vi "OC2 Read Sensor.vi"(0 "VISA resource name":refnum<visa-resource-name>, 1 "sensor report in":T1 {"Averaging" items=["Off", "On"]; "Unit" items=["deg C", "deg F", "deg K"]; "C coeff." format="%.2f"; "X coeff." format="%.2f"; "X2 coeff." format="%.2f"; "Sensor" items=["None", "PT100", "LM35", "LM50", "LM51", "LM60", "LM61", "Other"]}, 2 "error in (no error)":errorcluster, 5 "Enable":bool) -> (3 "dup VISA resource name":refnum<visa-resource-name>, 4 "sensor report out":T1 {"Averaging" items=["Off", "On"]; "Unit" items=["deg C", "deg F", "deg K"]; "C coeff." format="%.2f"; "X coeff." format="%.2f"; "X2 coeff." format="%.2f"; "Sensor" items=["None", "PT100", "LM35", "LM50", "LM51", "LM60", "LM61", "Other"]}, 6 "error out":errorcluster)   [LabVIEW 2009]
doc: "TCM Read Sensor.vi\n\nVI that reads the sensor information, accepts a cluster that contains the following variables:\nSensor type - PT100, LM35 etc\nx2, x, c coefficients - quadratic equation information\nUnit - unit of measure degrees c, f and kelvin\nAveraging - off no averaging of the signal, on signal is averaged\n\n\nCOPYRIGHT ELECTRON DYNAMICS LTD"
panel:
  in  "Command":string
  out "Rx string":string
  # "Read sensor data"
  # "V1.02"
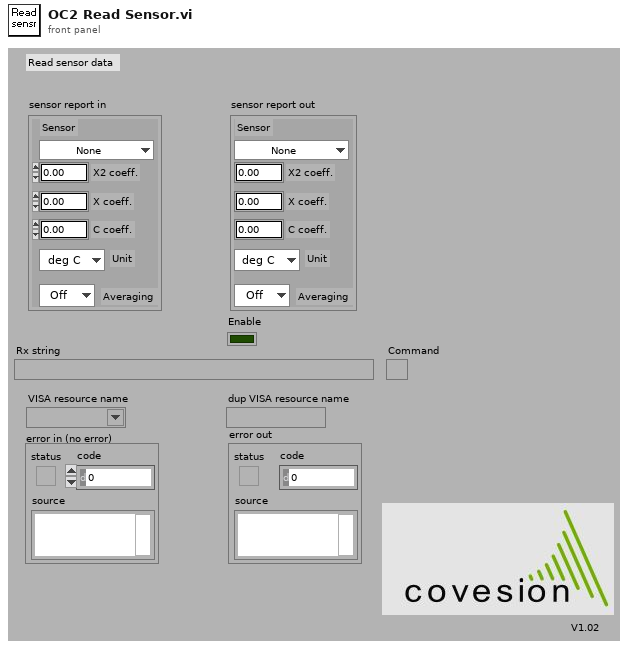
[diagram p1: front panel]
types:
  T1 = cluster{"Sensor":u16, "X2 coeff.":dbl, "X coeff.":dbl, "C coeff.":dbl, "Unit":u16, "Averaging":u16}
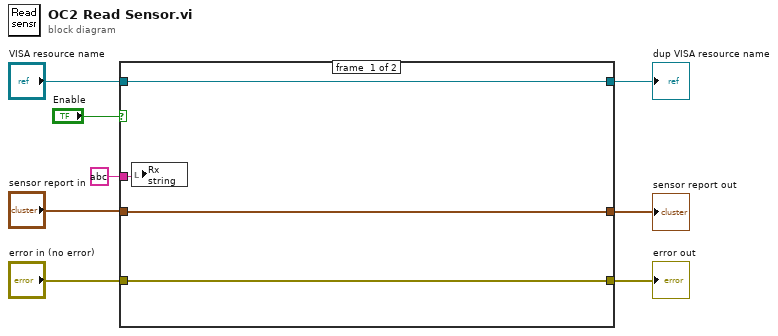
[diagram p0: block diagram]
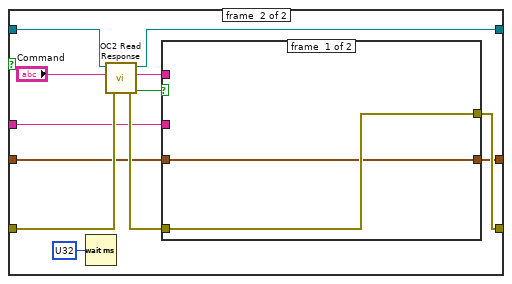
[diagram p2: hidden frame]
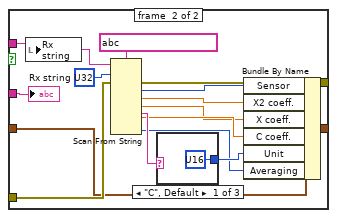
[diagram p3: hidden frame]
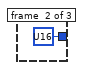
[diagram p4: hidden frame]
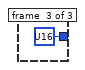
[diagram p5: hidden frame]
diagram:
  n1 = case shown="True" "Enable" {
    tunnel: "VISA resource name" -> [w12 w22]
    tunnel: [w12 w20] -> w7
    tunnel: "error in (no error)" -> [w11 w18]
    tunnel: [w11 w17] -> w5
    tunnel: [w10 w16] -> w3
    tunnel: "sensor report in" -> [w10 w15]
    tunnel: string ? ("Rx string") -> [w9 w14]
    frame #0 {
      n2 = local write "Rx string"(w9) -> ()
    }
    frame #1 {
      n3 = Wait (ms)(milliseconds to wait=u32 ?) -> ()  [unwired: 1 out]
      n4 = call "OC2 Read Response.vi"("error in (no error)"=w18, "Command"="Command", "VISA resource name"=w22) -> ("RX packet ok"=w21:bool, "error out"=w19:errorcluster, "output string"=w24:string, "dup VISA resource name"=w20:refnum<visa-resource-name>)  [unwired: 1 in]
      n5 = case shown="True" w21 {
        tunnel: w24 -> [_ w40]
        tunnel: w19 -> [w26 w31]
        tunnel: [w26 w32] -> w17
        tunnel: [w25 w30] -> w16
        tunnel: w15 -> [w25 w29]
        tunnel: w14 -> [_ w28]
        frame #0 {
        }
        frame #1 {
          n6 = local write "Rx string"(w40) -> ()
          n7 = Scan From String(format string=string ?, input string=w40, initial scan location=u32 ?, error in=w31) -> (error out=w32:errorcluster, output 1=w33:i32, output 2=w34:dbl, output 3=w35:dbl, output 4=w36:dbl, output 5=w39:string, output 6=w37:i32)  [unwired: 6 in, 2 out]
          n8 = case shown="\"C\", Default" w39 {
            tunnel: [u16 ? ("Averaging") u16 ? ("Averaging") u16 ? ("Averaging")] -> w38
            frame #0 {
            }
            frame #1 {
            }
            frame #2 {
            }
          }
          n9 = Bundle By Name(cluster=w29, "Sensor"=w33, "X2 coeff."=w34, "X coeff."=w35, "C coeff."=w36, "Unit"=w38, "Averaging"=w37) -> (w30:T1)
          "Rx string" <- w28
        }
      }
    }
  }
  "dup VISA resource name" <- w7
  "error out" <- w5
  "sensor report out" <- w3
